vi "PS_LCR_Command.vi"(11 "string":string) -> (0 "error out":errorcluster)   [LabVIEW 2011]
uses:
  PS_Global.vi
  <vilib>/Instr/_visa.llb/VISA Configure Serial Port (Instr).vi
panel:
  in  "baud rate":u32=115200
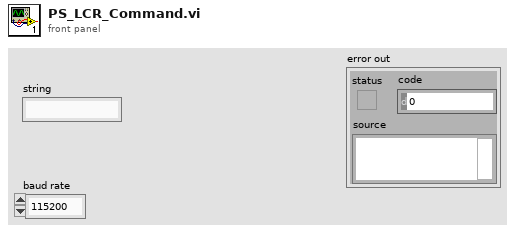
[diagram p1: front panel]
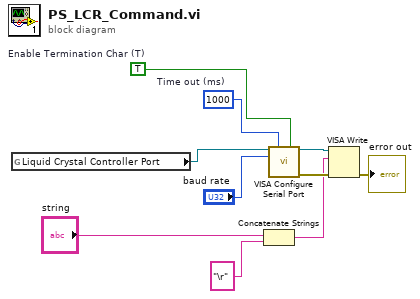
[diagram p0: block diagram]
diagram:
  w6 = TRUE  # Enable Termination Char (T)
  w9 = 1000  # Time out (ms)
  n1 = global read "PS_Global.vi" "Liquid Crystal Controller Port"() -> (w1:refnum<visa-resource-name>)
  n2 = Concatenate Strings("string", "\r") -> (w4:string)
  n3 = call-poly "VISA Configure Serial Port"("VISA resource name"=w1, "timeout (10sec)"=w9, "Enable Termination\nChar (T)"=w6, "baud rate (9600)"="baud rate") -> ("VISA resource name out"=w8:refnum<visa-resource-name>, "error out"=w7:errorcluster)  [unwired: 10 in]
  n4 = VISA Write(VISA resource name=w8, write buffer=w4, error in (no error)=w7) -> (error out=→"error out":errorcluster)  [unwired: 2 out]
